vi "Stirling Test.vi"() -> ()   [LabVIEW 2017]
panel:
  out "Debug _ \nApprox Percentage":dbl[](array[numeric])
  out "Index in That Array":dbl[](array[numeric])
  in  "Search Setting":T1={"Test Array"=[], "Max Value"=0.01, "Minimum Value"=0.008}
  in  "Test Range":dbl=150.0
  out "XY Graph":cluster{i32[], dbl[]}(graph)
  out "Output Cluster":T2
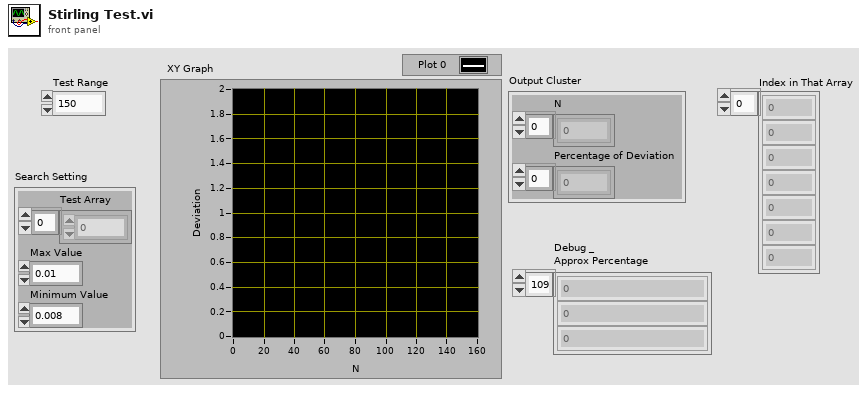
[diagram p1: front panel]
types:
  T1 = cluster{"Test Array":dbl[], "Max Value":dbl, "Minimum Value":dbl}
  T2 = cluster{"N":dbl[], "Percentage of Deviation":dbl[]}
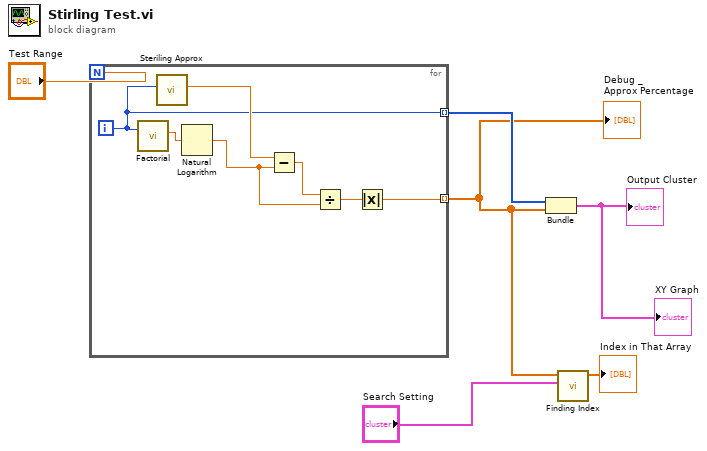
[diagram p0: block diagram]
diagram:
  n1 = for {
    N: "Test Range" -> [_]
    tunnel: [w10] -> w1 mode=indexing
    tunnel: [w9] -> w5 mode=indexing
    i -> [w9]
    n2 = call "Factorial.vi"("Factorial of Integer N"=w9) -> ("N!"=w8:dbl)  [unwired: 10 in]
    n3 = call "Steriling Approx.vi"("Large N"=w9) -> ("Approx."=w13:dbl)  [unwired: 10 in]
    n4 = Natural Logarithm(1:w8) -> (0:w7:dbl)
    n5 = Subtract(x=w13, y=w7) -> (x-y=w12:dbl)
    n6 = Divide(x=w12, y=w7) -> (x/y=w11:dbl)
    n7 = Absolute Value(x=w11) -> (abs(x)=w10:dbl)
  }
  "Debug _ \nApprox Percentage" <- w1
  n8 = Bundle(w5, w1) -> (→"Output Cluster" →"XY Graph":cluster{i32[], dbl[]})  [unwired: 1 in]
  n9 = call "Finding Index.vi"("Search Setting"="Search Setting", "Array to be Tested"=w1) -> ("Indexis taht falls in the range"=→"Index in That Array":dbl[])  [unwired: 9 in]
